vi "Switch Lat Long.vi"(1 "WP Lats and Longs for GIC":cluster{"WP Lats":dbl[], "WP Longs":dbl[]}) -> (0 "WP Lats and Longs switched":cluster{"WP Longs":dbl[], "WP Lats":dbl[]})   [LabVIEW 2014]
panel:
  # "Switch Lat and Long arrays in WP cluster for graph"
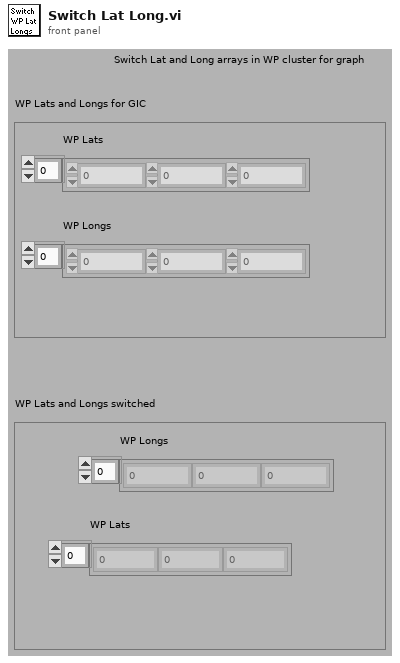
[diagram p1: front panel]
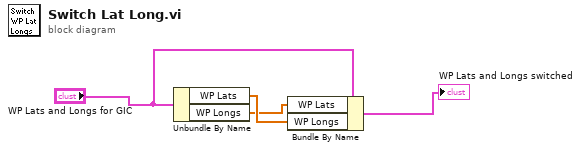
[diagram p0: block diagram]
diagram:
  n1 = Unbundle By Name("WP Lats and Longs for GIC") -> ("WP Lats"=w2:dbl[], "WP Longs"=w1:dbl[])
  n2 = Bundle By Name(cluster="WP Lats and Longs for GIC", "WP Lats"=w1, "WP Longs"=w2) -> (→"WP Lats and Longs switched":cluster{"WP Lats":dbl[], "WP Longs":dbl[]})
